vi "Exp data.vi"(6 "c":dbl, 8 "a":dbl, 9 "b":dbl, 10 "Number of points":i32, 11 "noise amplitude":dbl) -> (2 "X Array":i32[](array[numeric]), 3 "Y Array":dbl[](array[numeric]))   [LabVIEW 2023]
doc: "Creates a set of exponential data according to the model: y = a*exp(b*x) + c + noise."
uses:
  <vilib>/Analysis/NI_AALBase.lvlib
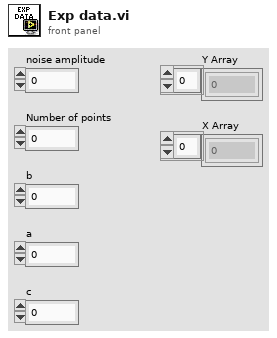
[diagram p1: front panel]
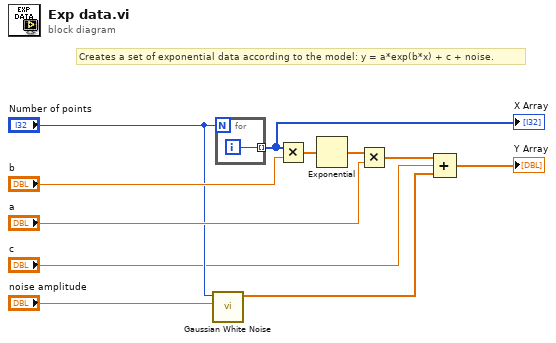
[diagram p0: block diagram]
diagram:
  # "Creates a set of exponential data according to the model: y = a*exp(b*x) + c + noise."
  n1 = call <vilib>:"Gaussian White Noise.vi"("standard deviation"="noise amplitude", "samples"="Number of points") -> ("Gaussian noise pattern"=w2:dbl[])  [unwired: 8 in, 1 out]
  n2 = for {
    N: "Number of points" -> [_]
    tunnel: [w12] -> w11 mode=indexing
    i -> [w12]
  }
  "X Array" <- w11
  n3 = Multiply(x=w11, y="b") -> (x*y=w7:dbl[])
  n4 = Exponential(1:w7) -> (0:w9:dbl[])
  n5 = Multiply(x=w9, y="a") -> (x*y=w4:dbl[])
  n6 = Compound Arithmetic op=ADD(w4, "c", w2) -> (→"Y Array":dbl[])
